vi "screw empty message.vi"   [LabVIEW 2015]
uses:
  Galobal variable_TI.vi
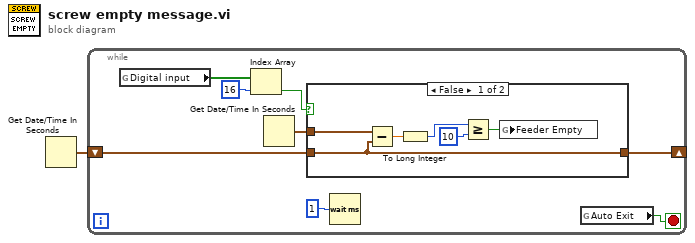
[diagram p0: block diagram]
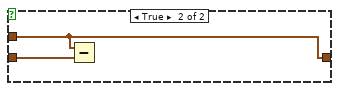
[diagram p2: hidden frame]
diagram:
  n1 = Get Date/Time In Seconds() -> (seconds since 1Jan1904=w1:timestamp)
  n2 = while {
    shift-right: [w3] -> _
    shift-left: w1 -> [w5]
    stop <- w6 stop-if-true
    n3 = global read "Galobal variable_TI.vi" "Digital input"() -> (w8:bool[])
    n4 = Index Array(array=w8, index=16) -> (element=w7:bool)
    n5 = Get Date/Time In Seconds() -> (seconds since 1Jan1904=w4:timestamp)
    n6 = case shown="False" w7 {
      tunnel: w5 -> [w13 w16]
      tunnel: w4 -> [w14 w17]
      tunnel: [w13 w17] -> w3
      frame False {
        n7 = Subtract(x=w14, y=w13) -> (x-y=w15:dbl)
        n8 = To Long Integer(number=w15) -> (32bit integer=w12:i32)
        n9 = Greater Or Equal?(x=w12, y=10) -> (x >= y?=w10:bool)
        n10 = global write "Galobal variable_TI.vi" "Feeder Empty"(w10) -> ()
      }
      frame True {
        n11 = Subtract(x=w17, y=w16) -> ()  [unwired: 1 out]
      }
    }
    n12 = Wait (ms)(milliseconds to wait=u32 1) -> ()  [unwired: 1 out]
    n13 = global read "Galobal variable_TI.vi" "Auto Exit"() -> (w6:bool)
  }
